vi "Polar_Arrays_To_Chart.vi"(10 "Direction":dbl[](array[numeric]), 11 "Magnitude":dbl[](array[numeric])) -> (0 "Y":dbl[](array[numeric]), 1 "X":dbl[](array[numeric]), 3 "Scan":cluster{"x":dbl, "y":dbl}[](array[cluster]))   [LabVIEW 2016, in "Hokuyo_URG.lvlib"]
uses:
  Hokuyo_URG.lvlib
  <vilib>/ptbypt/NI_PtbyPt.lvlib
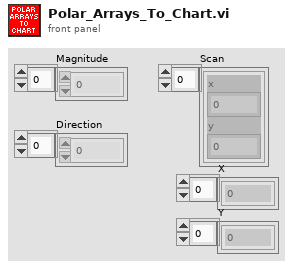
[diagram p1: front panel]
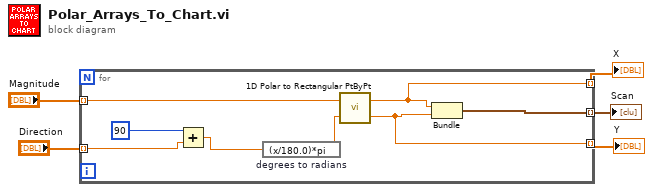
[diagram p0: block diagram]
diagram:
  n1 = for {
    tunnel: "Magnitude" -> [w13] mode=indexing
    tunnel: "Direction" -> [w10] mode=indexing
    tunnel: [w12] -> w5 mode=indexing
    tunnel: [w7] -> w2 mode=indexing
    tunnel: [w6] -> w1 mode=indexing
    n2 = Add(x=90, y=w10) -> (x+y=w8:dbl)
    n3 = expression code="(x/180.0)*pi" "degrees to radians"(w8) -> (w11:dbl)
    n4 = call <vilib>:"1D Polar to Rectangular PtByPt.vi"("phase"=w11, "magnitude"=w13) -> ("y"=w6:dbl, "x"=w7:dbl)
    n5 = Bundle("x"=w7, "y"=w6) -> (w12:cluster{"x":dbl, "y":dbl})  [unwired: 1 in]
  }
  "Scan" <- w5
  "X" <- w2
  "Y" <- w1
